vi "Extract Varient (static).vi"(7 "Copy":bool caption="Copy data instead of extracting", 8 "error in (no error)":errorcluster, 11 "Interprocess Message in":refnum<class "MSG.lvclass">) -> (0 "error out":errorcluster, 1 "Varient":variant, 2 "Label":string, 3 "Message (data extracted)":refnum<class "MSG.lvclass">)   [LabVIEW 2011, in "Messenging.lvlib" / "MSG.lvclass"]
uses:
  TextVarientMessage/MSG.lvclass
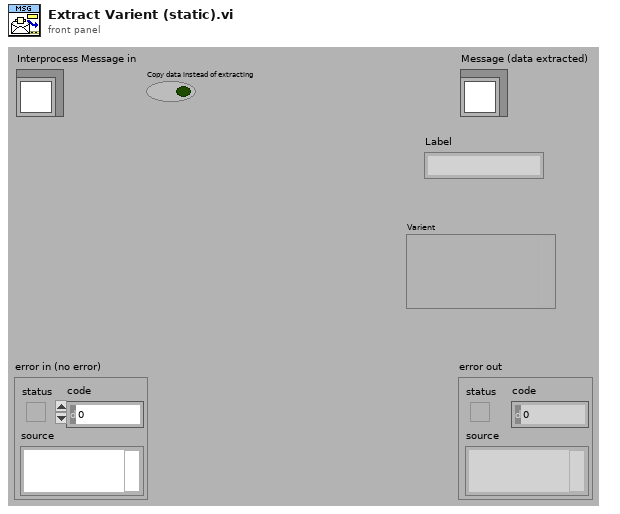
[diagram p1: front panel]
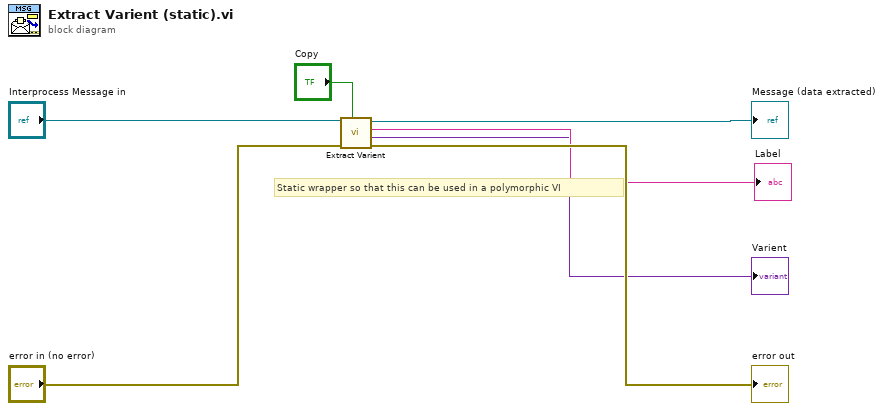
[diagram p0: block diagram]
diagram:
  # "Static wrapper so that this can be used in a polymorphic VI"
  n1 = call-dynamic "Extract Varient.vi"("Copy"="Copy", "error in (no error)"="error in (no error)", "Message"="Interprocess Message in") -> ("error out"=→"error out":errorcluster, "Varient"=→"Varient":variant, "Label"=→"Label":string, "Message"=→"Message (data extracted)":refnum<class "MSG.lvclass">)  [unwired: 5 out]
